vi "Cluster Make Typedef Elements Info.vi"(7 "skip first typedef?":bool, 8 "error in (no error)":errorcluster, 10 "ClusterConstant refnum":refnum<vi>, 11 "Terminal in":refnum<vi>) -> (0 "error out":errorcluster, 1 "is typedef?":bool, 2 "Cluster elements datatypes":string[](array[string]), 3 "Cluster elements names":string[](array[string]), 4 "typedef name":string)   [LabVIEW 2014]
doc: "Return info about cluster elements, as input use Terminal or ClusterConstant (use just one of them)\nIf wired Cluster Constant refnum returns names and datatypes of elements inside cluster. If element has no label, it's returned default name \"item0\" or \"item1\" or ... \"itemN\" which will be also used in generated code.\nIf wired Terminal then is used to get names and datatypes of cluster, it will programmaticaly creates cluster constant on diagram, inspects its elements, removes it and return elements info.\nThis VI return elements datatypes, if inside cluster is another cluster it returns for that item its typedefinition ie.:\n struct{\n struct{int A; String B; someTypedefStructName C;} itemName;\n }"
uses:
  TranscriptorBasicObject.lvclass
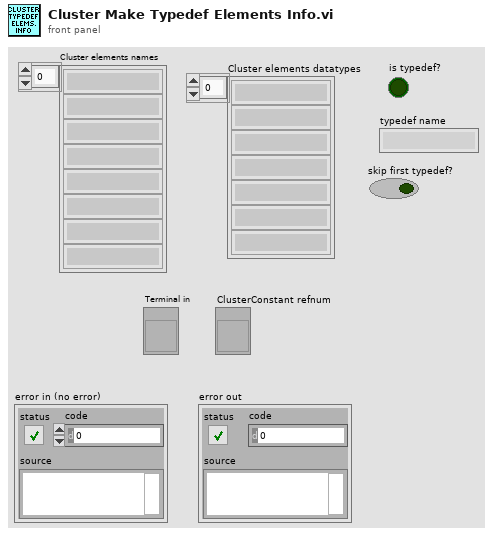
[diagram p1: front panel]
types:
  T1 = enum32{"not a typedef", "typedef", "strict typedef", "class private data"}[]
  T2 = enum32{"not a typedef", "typedef", "strict typedef", "class private data"}
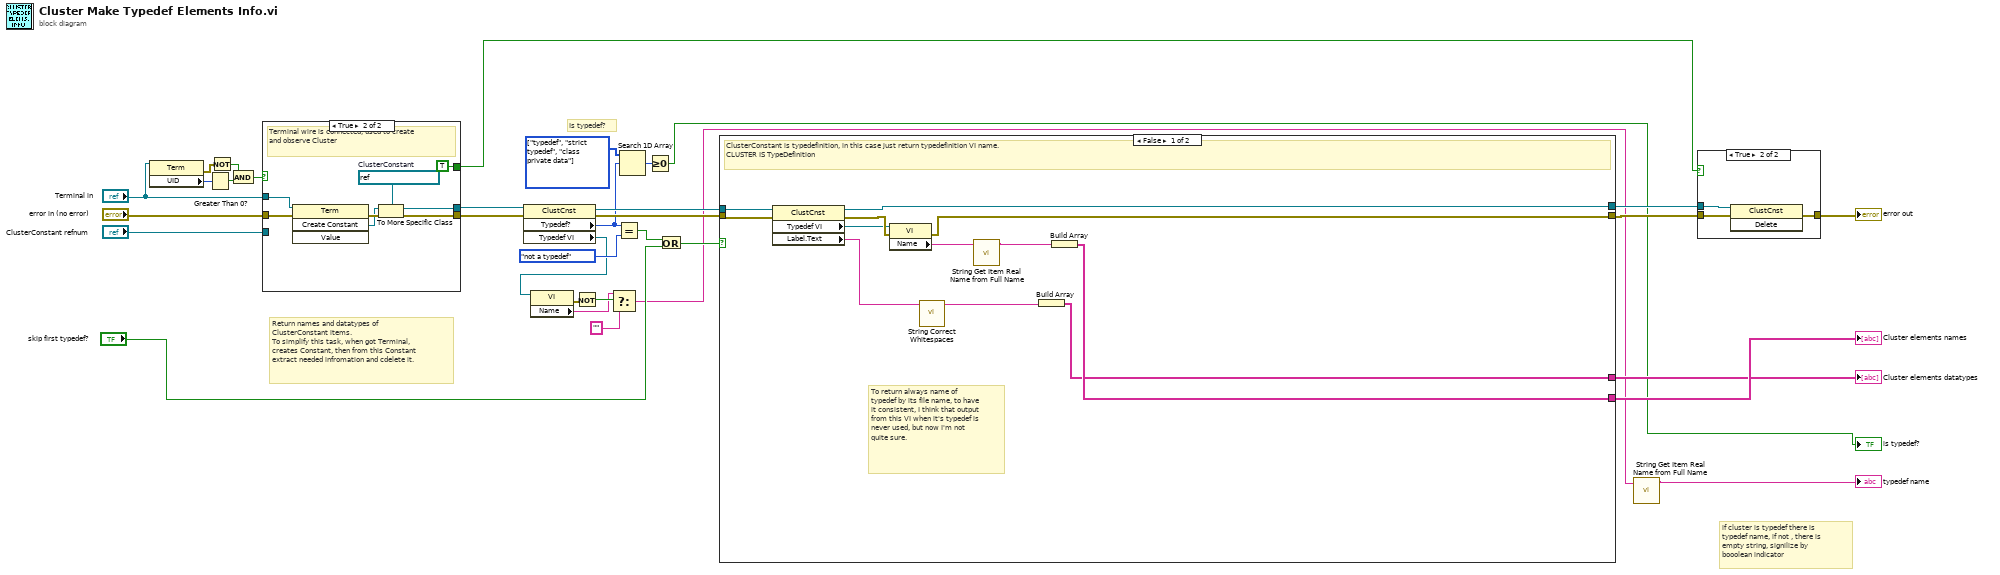
[diagram p0: block diagram]
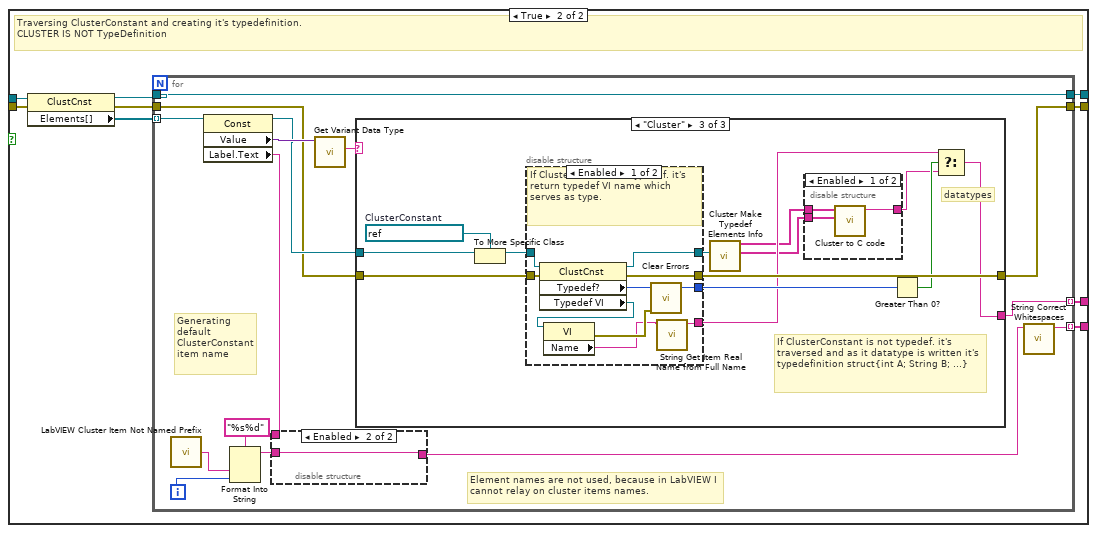
[diagram p2: hidden frame]
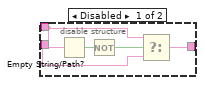
[diagram p3: hidden frame]
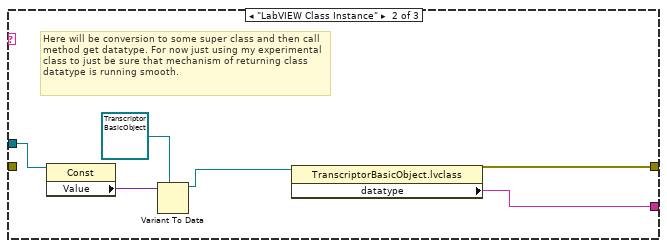
[diagram p5: hidden frame]
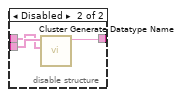
[diagram p6: hidden frame]
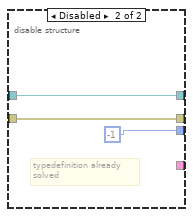
[diagram p7: hidden frame]
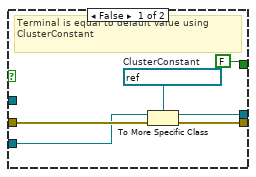
[diagram p9: hidden frame]
diagram:
  w13 = T1 [enum."typedef", enum."strict typedef", enum."class private data"] items=["not a typedef", "typedef", "strict typedef", "class private data"]
  # "Is typedef?"
  # "if cluster is typedef there is typedef name, if not , there is empty string, signilize by booolean indicator"
  # "Return names and datatypes of ClusterConstant items.\nTo simplify this task, when got Terminal, creates Constant, then from this Constant extract needed infromation and cdelete it."
  n1 = property class="Term"(reference="Terminal in") -> (error out=w21:errorcluster, "UID"=w23:i32)  [unwired: 1 in, 1 out]
  n2 = Greater Than 0?(x=w23) -> (x > 0?=w22:bool)
  n3 = Not(x=w21) -> (.not. x?=w20:bool)
  n4 = And(x=w20, y=w22) -> (x .and. y?=w19:bool)
  n5 = case shown="True" w19 {
    tunnel: [w37 w47] -> w27
    tunnel: "error in (no error)" -> [w36 w45]
    tunnel: [w38 w43] -> w17
    tunnel: "Terminal in" -> [_ w41]
    tunnel: [FALSE TRUE] -> w26
    tunnel: "ClusterConstant refnum" -> [w34 _]
    frame False {
      w39 = refnum<vi> refnum  # ClusterConstant
      # "Terminal is equal to default value using ClusterConstant"
      n6 = To More Specific Class(target class=w39, reference=w34, error in=w36) -> (specific class reference=w38:refnum<vi>, error out=w37:errorcluster)
    }
    frame True {
      w42 = refnum<vi> refnum  # ClusterConstant
      # "Terminal wire is connected, used to create and observe Cluster"
      n7 = invoke on="Invoke Node" class="Term" method="Create Constant"(reference=w41, error in=w45) -> (error out=w46:errorcluster, "Create Constant"=w44:refnum<vi>)  [unwired: 2 in, 2 out]
      n8 = To More Specific Class(target class=w42, reference=w44, error in=w46) -> (specific class reference=w43:refnum<vi>, error out=w47:errorcluster)
    }
  }
  n9 = property on="Property Node" class="ClustCnst"(reference=w17, error in=w27) -> (reference out=w16:refnum<vi>, error out=w15:errorcluster, "Typedef?"=w12:T2, "Typedef VI"=w7:refnum<vi>)
  n10 = property on="Property Node" class="VI"(reference=w7) -> (error out=w6:errorcluster, "Name"=w4:string)  [unwired: 1 in, 1 out]
  n11 = Not(x=w6) -> (.not. x?=w5:bool)
  n12 = Select(t=w4, s=w5, f="") -> (s? t:f=w1:string)
  n13 = Equal?(x=w12, y=T2."not a typedef" ("Is Typedef?")) -> (x = y?=w10:bool)
  n14 = Search 1D Array(1D array=w13, element=w12) -> (index of element=w11:i32)  [unwired: 1 in]
  n15 = Greater Or Equal To 0?(x=w11) -> (x >= 0?=→"is typedef?":bool)
  n16 = Or(x=w10, y="skip first typedef?") -> (x .or. y?=w9:bool)
  n17 = case shown="False" w9 {
    tunnel: [w55 w68] -> w32
    tunnel: w15 -> [w58 w66]
    tunnel: w16 -> [w59 w64]
    tunnel: [w57 w62] -> w30
    tunnel: [w54 w61] -> w29
    tunnel: [w50 w60] -> w28
    frame False {
      # "To return always name of typedef by its file name, to have it consistent, I think that output from this VI when it's typedef is never used, but now I'm not quite sure."
      # "ClusterConstant is typedefinition, in this case just return typedefinition VI name.\nCLUSTER IS TypeDefinition"
      n18 = property on="Property Node" class="ClustCnst"(reference=w59, error in=w58) -> (reference out=w57:refnum<vi>, error out=w56:errorcluster, "Typedef VI"=w52:refnum<vi>, "Label.Text"=w53:string)
      n19 = property on="Property Node" class="VI"(reference=w52, error in=w56) -> (error out=w55:errorcluster, "Name"=w48:string)  [unwired: 1 out]
      n20 = call "String Correct Whitespaces.vi"("String in"=w53) -> ("String out"=w51:string)  [unwired: 10 in]
      n21 = call "String Get Item Real Name from Full Name.vi"("Full name with lib/class prefix"=w48) -> ("real short name"=w49:string)  [unwired: 10 in]
      n22 = Build Array(w51) -> (w50:string[])
      n23 = Build Array(w49) -> (w54:string[])
    }
    frame True {
      # "Traversing ClusterConstant and creating it's typedefinition.\nCLUSTER IS NOT TypeDefinition"
      n24 = property on="Property Node" class="ClustCnst"(reference=w64, error in=w66) -> (reference out=w63:refnum<vi>, error out=w67:errorcluster, "Elements[]"=w65:refnum<vi>[])
      n25 = for {
        tunnel: w65 -> [w83] mode=indexing
        tunnel: w67 -> [w69]
        tunnel: [w71] -> w68
        tunnel: w63 -> [w77]
        tunnel: [w77] -> w62
        tunnel: [w70] -> w60 mode=indexing
        tunnel: [w76] -> w61 mode=indexing
        i -> [w80]
        # "Element names are not used, because in LabVIEW I cannot relay on cluster items names."
        # "Generating default ClusterConstant item name"
        n26 = call "LabVIEW Cluster Item Not Named Prefix.vi"() -> ("not named cluster item prefix"=w79:string)
        n27 = property class="Const"(reference=w83) -> (reference out=w72:refnum<vi>, "Value"=w73:variant, "Label.Text"=w78:string)  [unwired: 1 in, 1 out]
        n28 = Format Into String(format string="%s%d", w79, w80) -> (resulting string=w81:string)  [unwired: 2 in, 1 out]
        n29 = disable-structure shown="Enabled" {
          disable-tunnel: w81 -> [w86 w89]
          disable-tunnel: w78 -> [w85 _]
          disable-tunnel: [w84 w89] -> w75
          frame Disabled {
            n30 = Empty String/Path?(string/path=w85) -> (empty?=w88:bool)
            n31 = Not(x=w88) -> (.not. x?=w87:bool)
            n32 = Select(t=w85, s=w87, f=w86) -> (s? t:f=w84:string)
          }
          frame Enabled {
          }
        }
        n33 = call "Get Variant Data Type.vi"("Variant in"=w73) -> ("first data type"=w74:string)  [unwired: 9 in, 1 out]
        n34 = case shown="\"Cluster\"" w74 {
          selector: w74 -> [w90 _ _]
          tunnel: w72 -> [_ w95 w100]
          tunnel: w69 -> [w91 _ w109]
          tunnel: [w91 w96 w107] -> w71
          tunnel: [w90 w97 w106] -> w70
          frame Default {
          }
          frame "LabVIEW Class Instance" {
            # "Here will be conversion to some super class and then call method get datatype. For now just using my experimental class to just be sure that mechanism of returning class datatype is running smooth."
            n35 = property class="Const"(reference=w95) -> ("Value"=w94:variant)  [unwired: 1 in, 2 out]
            n36 = Variant To Data(type=refnum<class "TranscriptorBasicObject.lvclass"> refnum ("TranscriptorBasicObject.lvclass"), Variant=w94) -> (data=w93:refnum<class "TranscriptorBasicObject.lvclass">)  [unwired: 1 in, 1 out]
            n37 = property class="TranscriptorBasicObject.lvclass"(reference=w93) -> (error out=w96:errorcluster, "datatype"=w97:string)  [unwired: 1 in, 1 out]
          }
          frame "Cluster" {
            w110 = refnum<vi> refnum  # ClusterConstant
            # "If ClusterConstant is not typedef. it's traversed and as it datatype is written it's typedefinition struct{int A; String B; ...}"
            # "datatypes"
            n38 = To More Specific Class(target class=w110, reference=w100) -> (specific class reference=w99:refnum<vi>)  [unwired: 1 in, 1 out]
            n39 = disable-structure shown="Enabled" {
              disable-tunnel: w109 -> [w125 w128]
              disable-tunnel: [w124 -1] -> w108
              disable-tunnel: [w121 w128] -> w107
              disable-tunnel: [w118 _] -> w104
              disable-tunnel: w99 -> [w120 w126]
              disable-tunnel: [w119 w126] -> w98
              frame Enabled {
                # "If ClusterConstant is typedef. it's return typedef VI name which serves as type."
                n40 = property class="ClustCnst"(reference=w120, error in=w125) -> (reference out=w119:refnum<vi>, error out=w121:errorcluster, "Typedef?"=w124:T2, "Typedef VI"=w122:refnum<vi>)
                n41 = property class="VI"(reference=w122) -> (error out=w123:errorcluster, "Name"=w117:string)  [unwired: 1 in, 1 out]
                n42 = call <vilib>:"Clear Errors.vi"("error in (no error)"=w123) -> ()  [unwired: 5 in, 2 out]
                n43 = call "String Get Item Real Name from Full Name.vi"("Full name with lib/class prefix"=w117) -> ("real short name"=w118:string)  [unwired: 10 in]
              }
              frame Disabled {
                # "typedefinition already\nsolved"
              }
            }
            n44 = call "Cluster Make Typedef Elements Info.vi"("ClusterConstant refnum"=w98) -> ("Cluster elements datatypes"=w102:string[], "Cluster elements names"=w103:string[])  [unwired: 6 in, 3 out]
            n45 = disable-structure shown="Enabled" {
              disable-tunnel: w103 -> [w113 w115]
              disable-tunnel: w102 -> [w112 w116]
              disable-tunnel: [w111 w114] -> w101
              frame Enabled {
                n46 = call "Cluster to C code.vi"("Cluster elements datatypes"=w112, "Cluster elements names"=w113) -> ("C code"=w111:string)  [unwired: 9 in]
              }
              frame Disabled {
                n47 = call "Cluster Generate Datatype Name.vi"("Cluster elements names"=w115, "Cluster elements datatypes"=w116) -> ("generated datatype name"=w114:string)  [unwired: 9 in]
              }
            }
            n48 = Greater Than 0?(x=w108) -> (x > 0?=w105:bool)
            n49 = Select(t=w104, s=w105, f=w101) -> (s? t:f=w106:string)
          }
        }
        n50 = call "String Correct Whitespaces.vi"("String in"=w75) -> ("String out"=w76:string)  [unwired: 10 in]
      }
    }
  }
  "Cluster elements datatypes" <- w28
  "Cluster elements names" <- w29
  n51 = call "String Get Item Real Name from Full Name.vi"("Full name with lib/class prefix"=w1) -> ("real short name"=→"typedef name":string)  [unwired: 10 in]
  n52 = case shown="True" w26 {
    tunnel: [w129 w132] -> w33
    tunnel: w32 -> [w129 w131]
    tunnel: w30 -> [_ w130]
    frame False {
    }
    frame True {
      n53 = invoke on="Invoke Node" class="ClustCnst" method="Delete"(reference=w130, error in=w131) -> (error out=w132:errorcluster)  [unwired: 1 in, 2 out]
    }
  }
  "error out" <- w33
